vi "Joystick Drive.vi"(0 "Right Side?":bool, 1 "Turn?":bool, 2 "Fire?":bool) -> (6 "Aligned?":bool, 8 "Bridge Mode?":bool, 9 "Viewer Select":T1(ring)=enum."Ball Camera")   [LabVIEW 2011]
uses:
  Team Code/Robot Global Data.vi
panel:
  in  "Power Factor":dbl=2.0
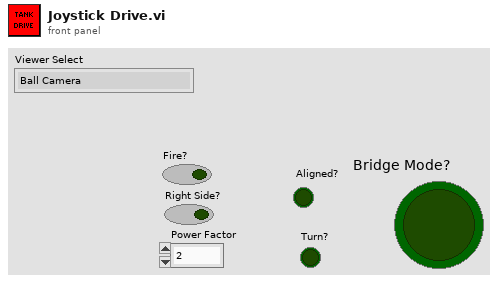
[diagram p1: front panel]
types:
  T1 = enum32{"Target Camera", "Target Camera Mask", "Ball Camera", "Kinect Skeleton"}
  T2 = typedef "WPI_JoystickButtonState.ctl" = cluster{"Button 1":bool, "Button 2":bool, "Button 3":bool, "Button 4":bool, "Button 5":bool, "Button 6":bool, "Button 7":bool, "Button 8":bool, "Button 9":bool, "Button 10":bool, "Button 11":bool, "Button 12":bool}
  T3 = cluster{"Buttons":T2, "Axes":cluster{"axis 1 (x)":dbl, "axis 2 (y)":dbl, "axis 3 (throttle)":dbl, "axis 4":dbl, "axis 5":dbl, "axis 6":dbl}}
  T4 = cluster{"Position":cluster{"X Angle":dbl, "Raw Y":dbl, "Raw X":dbl}, "Distance (ft)":dbl, "BB Angle":dbl}
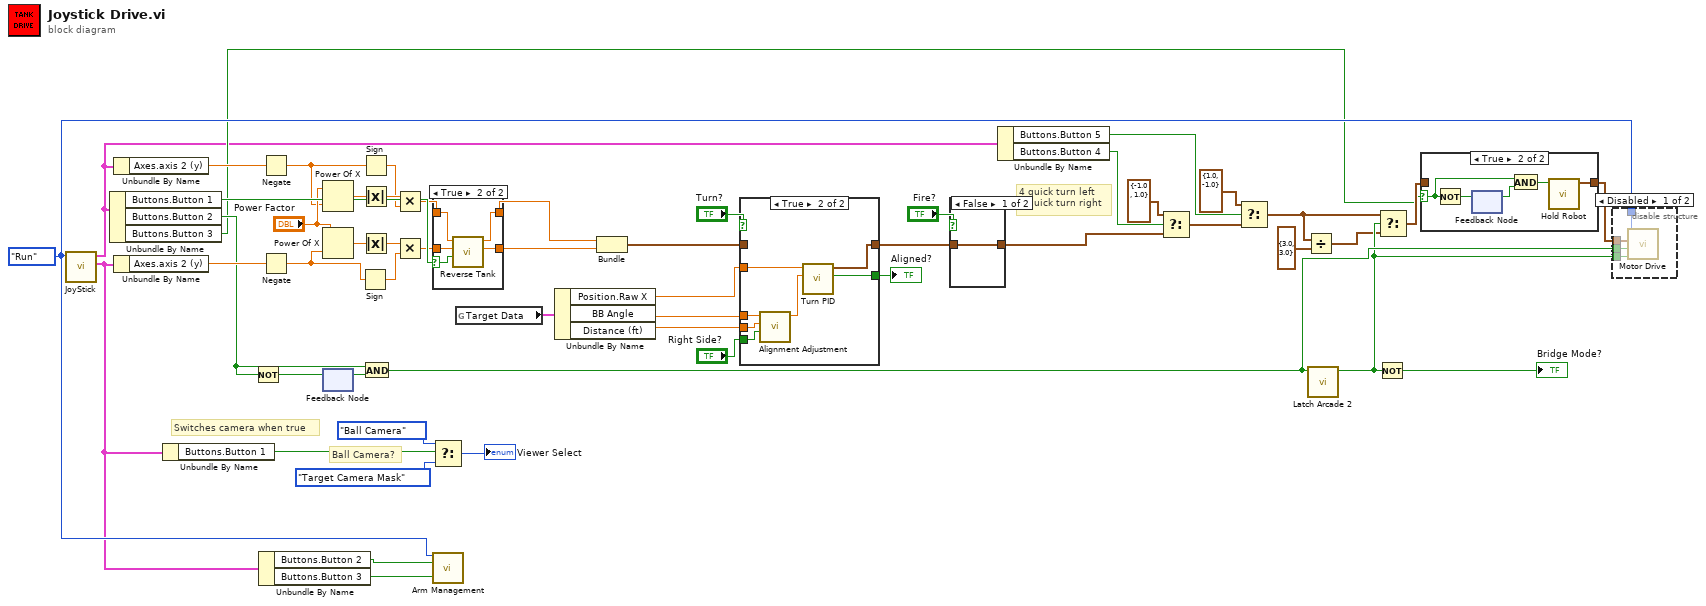
[diagram p0: block diagram]
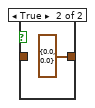
[diagram p5: hidden frame]
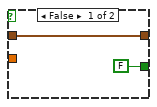
[diagram p6: hidden frame]
diagram:
  w11 = enum16{"Init", "Run", "End"}."Run" ("Enum")
  # "Switches camera when true"
  # "Ball Camera?"
  # "4 quick turn left\n5 quick turn right"
  n1 = call "JoyStick.vi"("Enum"=w11) -> ("JoyStick 2"=w10:T3, "JoyStick 1"=w1:T3)  [unwired: 7 in, 2 out]
  n2 = Unbundle By Name(w1) -> ("Buttons.Button 1"=w43:bool, "Buttons.Button 2"=w3:bool, "Buttons.Button 3"=w2:bool)
  n3 = Unbundle By Name(w1) -> ("Axes.axis 2 (y)"=w53:dbl)
  n4 = Unbundle By Name(w10) -> ("Axes.axis 2 (y)"=w52:dbl)
  n5 = Unbundle By Name(w10) -> ("Buttons.Button 1"=w6:bool)
  n6 = Not(x=w3) -> (.not. x?=w45:bool)
  n7 = Unbundle By Name(w10) -> ("Buttons.Button 2"=w13:bool, "Buttons.Button 3"=w12:bool)
  n8 = Negate(x=w53) -> (-x=w32:dbl)
  n9 = Negate(x=w52) -> (-x=w25:dbl)
  n10 = Power Of X(1:w32, 2:"Power Factor") -> (0:w29:dbl)
  n11 = Power Of X(1:w25, 2:"Power Factor") -> (0:w24:dbl)
  n12 = feedback #1() -> (w44:bool)  [unwired: 1 in]
  n13 = feedback-in #1(w45) -> ()
  n14 = Sign(1:w25) -> (0:w26:dbl)
  n15 = Sign(1:w32) -> (0:w30:dbl)
  n16 = Absolute Value(x=w29) -> (abs(x)=w31:dbl)
  n17 = Absolute Value(x=w24) -> (abs(x)=w27:dbl)
  n18 = And(x=w3, y=w44) -> (x .and. y?=w37:bool)
  n19 = Multiply(x=w31, y=w30) -> (x*y=w28:dbl)
  n20 = Multiply(x=w27, y=w26) -> (x*y=w23:dbl)
  n21 = case shown="True" w43 {
    selector: w43 -> [_ w60]
    tunnel: w23 -> [w55 w59]
    tunnel: w28 -> [w54 w58]
    tunnel: [w54 w57] -> w42
    tunnel: [w55 w56] -> w41
    frame False {
    }
    frame True {
      n22 = call "Reverse Tank.vi"("Toggle Button"=w60, "Right Motor"=w59, "Left Motor"=w58) -> ("Right Motor"=w56:dbl, "Left Motor"=w57:dbl)  [unwired: 7 in]
    }
  }
  n23 = Select(t=T1."Ball Camera" ("Viewer Select"), s=w6, f=T1."Target Camera Mask" ("Viewer Select")) -> (s? t:f=→"Viewer Select":T1)
  n24 = call "Arm Management.vi"("Enum"=w11, "Up Button"=w13, "Down Button"=w12) -> ()  [unwired: 13 in]
  n25 = global read "Robot Global Data.vi" "Target Data"() -> (w50:T4)
  n26 = Unbundle By Name(w50) -> ("Position.Raw X"=w49:dbl, "BB Angle"=w14:dbl, "Distance (ft)"=w15:dbl)
  n27 = Bundle("Left Motor"=w42, "Right Motor"=w41) -> (w51:cluster{"Left Motor":dbl, "Right Motor":dbl})  [unwired: 1 in]
  n28 = case shown="True" "Turn?" {
    tunnel: [w62 w68] -> w47
    tunnel: w51 -> [w62 _]
    tunnel: w49 -> [_ w69]
    tunnel: w14 -> [_ w67]
    tunnel: w15 -> [_ w66]
    tunnel: "Right Side?" -> [_ w65]
    tunnel: [FALSE w63] -> w39
    frame False {
    }
    frame True {
      n29 = call "Alignment Adjustment.vi"("Right Side of Field?"=w65, "Distance"=w66, "BB Angle"=w67) -> ("X Setpoint"=w64:dbl)  [unwired: 8 in]
      n30 = call "Turn PID.vi"("Setpoint X"=w64, "Current X"=w69) -> ("Aligned?"=w63:bool, "Motor Out"=w68:cluster{"output":dbl, dbl})  [unwired: 8 in]
    }
  }
  "Aligned?" <- w39
  n31 = case shown="False" "Fire?" {
    tunnel: w47 -> [w70 _]
    tunnel: [w70 cluster{"output":dbl, dbl} {"output"=0.0, 0.0} ("Motor Out")] -> w22
    frame False {
    }
    frame True {
    }
  }
  n32 = Unbundle By Name(w1) -> ("Buttons.Button 5"=w16:bool, "Buttons.Button 4"=w17:bool)
  n33 = Select(t=cluster{"output":dbl, "Right Motor":dbl} {"output"=-1.0, "Right Motor"=1.0}, s=w17, f=w22) -> (s? t:f=w20:cluster{"output":dbl, "Right Motor":dbl})
  n34 = Select(t=cluster{"output":dbl, "Right Motor":dbl} {"output"=1.0, "Right Motor"=-1.0}, s=w16, f=w20) -> (s? t:f=w18:cluster{"output":dbl, "Right Motor":dbl})
  n35 = Divide(x=w18, y=cluster{"output":dbl, "Right Motor":dbl} {"output"=3.0, "Right Motor"=3.0}) -> (x/y=w34:cluster{"output":dbl, "Right Motor":dbl})
  n36 = call "Latch Arcade 2.vi"("Input"=w37) -> ("Latched"=w35:bool)  [unwired: 10 in]
  n37 = Not(x=w35) -> (.not. x?=→"Bridge Mode?":bool)
  n38 = Select(t=w18, s=w35, f=w34) -> (s? t:f=w5:cluster{"output":dbl, "Right Motor":dbl})
  n39 = case shown="True" w2 {
    selector: w2 -> [_ w75]
    tunnel: w5 -> [w72 _]
    tunnel: [w72 w77] -> w4
    frame False {
    }
    frame True {
      n40 = Not(x=w75) -> (.not. x?=w74:bool)
      n41 = feedback-in #2(w74) -> ()
      n42 = feedback #2() -> (w76:bool)  [unwired: 1 in]
      n43 = And(x=w75, y=w76) -> (x .and. y?=w73:bool)
      n44 = call "Hold Robot.vi"("Reset Encoders?"=w73) -> ("Speed Output"=w77:cluster{"output":dbl, "output":dbl})  [unwired: 10 in]
    }
  }
  n45 = disable-structure shown="Disabled" {
    disable-tunnel: w37 -> [w81 _]
    disable-tunnel: w35 -> [w80 _]
    disable-tunnel: w11 -> [w79 _]
    disable-tunnel: w4 -> [w78 _]
    frame Disabled {
      n46 = call "Motor Drive.vi"("Coast?"=w80, "Change Mode?"=w81, "Motor Input"=w78, "Enum"=w79) -> ()  [unwired: 8 in]
    }
    frame Enabled {
    }
  }
